vi "EllipseAxes.vi"(3 "error in (no error)":errorcluster, 4 "input cluster":T1) -> (0 "error out":errorcluster, 1 "Minor axis":dbl, 2 "Major axis":dbl)   [LabVIEW 2015]
uses:
  <vilib>/vision/NI_Vision_Development_Module.lvlib
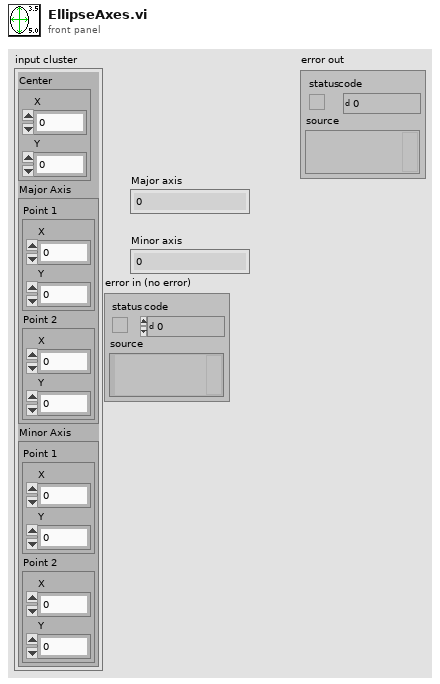
[diagram p1: front panel]
types:
  T1 = cluster{"Center":cluster{"X":sgl, "Y":sgl}, "Major Axis":cluster{"Point 1":cluster{"X":sgl, "Y":sgl}, "Point 2":cluster{"X":sgl, "Y":sgl}}, "Minor Axis":cluster{"Point 1":cluster{"X":sgl, "Y":sgl}, "Point 2":cluster{"X":sgl, "Y":sgl}}}
  T2 = cluster{"Point 1":cluster{"X":sgl, "Y":sgl}, "Point 2":cluster{"X":sgl, "Y":sgl}}
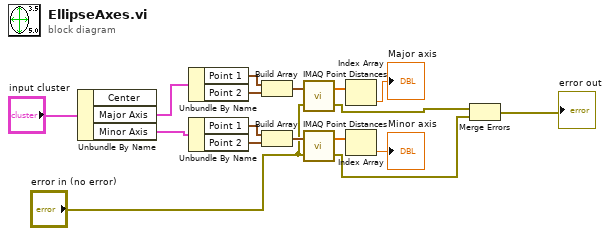
[diagram p0: block diagram]
diagram:
  n1 = Unbundle By Name("input cluster") -> ("Major Axis"=w17:T2, "Minor Axis"=w7:T2)  [unwired: 1 out]
  n2 = Unbundle By Name(w17) -> ("Point 1"=w16:cluster{"X":sgl, "Y":sgl}, "Point 2"=w15:cluster{"X":sgl, "Y":sgl})
  n3 = Unbundle By Name(w7) -> ("Point 1"=w11:cluster{"X":sgl, "Y":sgl}, "Point 2"=w10:cluster{"X":sgl, "Y":sgl})
  n4 = Build Array(w16, w15) -> (w14:cluster{"X":sgl, "Y":sgl}[])
  n5 = Build Array(w11, w10) -> (w9:cluster{"X":sgl, "Y":sgl}[])
  n6 = call "IMAQ Point Distances"("Points"=w14, "error in (no error)"="error in (no error)") -> ("Distances"=w13:sgl[], "error out"=w2:errorcluster)  [unwired: 3 in]
  n7 = call "IMAQ Point Distances"("Points"=w9, "error in (no error)"="error in (no error)") -> ("Distances"=w8:sgl[], "error out"=w3:errorcluster)  [unwired: 3 in]
  n8 = Index Array(array=w13) -> (element=→"Major axis":sgl)  [unwired: 1 in]
  n9 = Index Array(array=w8) -> (element=→"Minor axis":sgl)  [unwired: 1 in]
  n10 = Merge Errors(w2, w3) -> (→"error out":errorcluster)
